vi "Initialise Teapot.vi"(8 "error in (no error)":errorcluster, 11 "Resource Directory":path) -> (0 "error out":errorcluster, 3 "Teapot":T1 {"Triangles"."Vertex 3"."UV"."v" min=0 max=1 step=0.1; "Triangles"."Vertex 3"."UV"."u" min=0 max=1 step=0.1; "Triangles"."Vertex 2"."UV"."v" min=0 max=1 step=0.1; "Triangles"."Vertex 2"."UV"."u" min=0 max=1 step=0.1; "Triangles"."Vertex 1"."UV"."v" min=0 max=1 step=0.1; "Triangles"."Vertex 1"."UV"."u" min=0 max=1 step=0.1})   [LabVIEW 2022 SP3, in "Application.lvlib" / "Scene.lvclass"]
uses:
  Scene.lvclass
  Libraries/3D/Object.ctl
  Libraries/3D/Vector 3D.ctl
  Libraries/3D/Transform.ctl
  <userlib>/_OpenG.lib/file/file.llb/Convert File Extension (Path)__ogtk.vi
  Scene.lvclass/Scene.ctl
  Libraries/3D/3D.lvlib
  Libraries/Raster/UV.ctl
  Libraries/Raster/Raster.lvlib
  Libraries/3D/Vertex.ctl
  Libraries/3D/Triangle.ctl
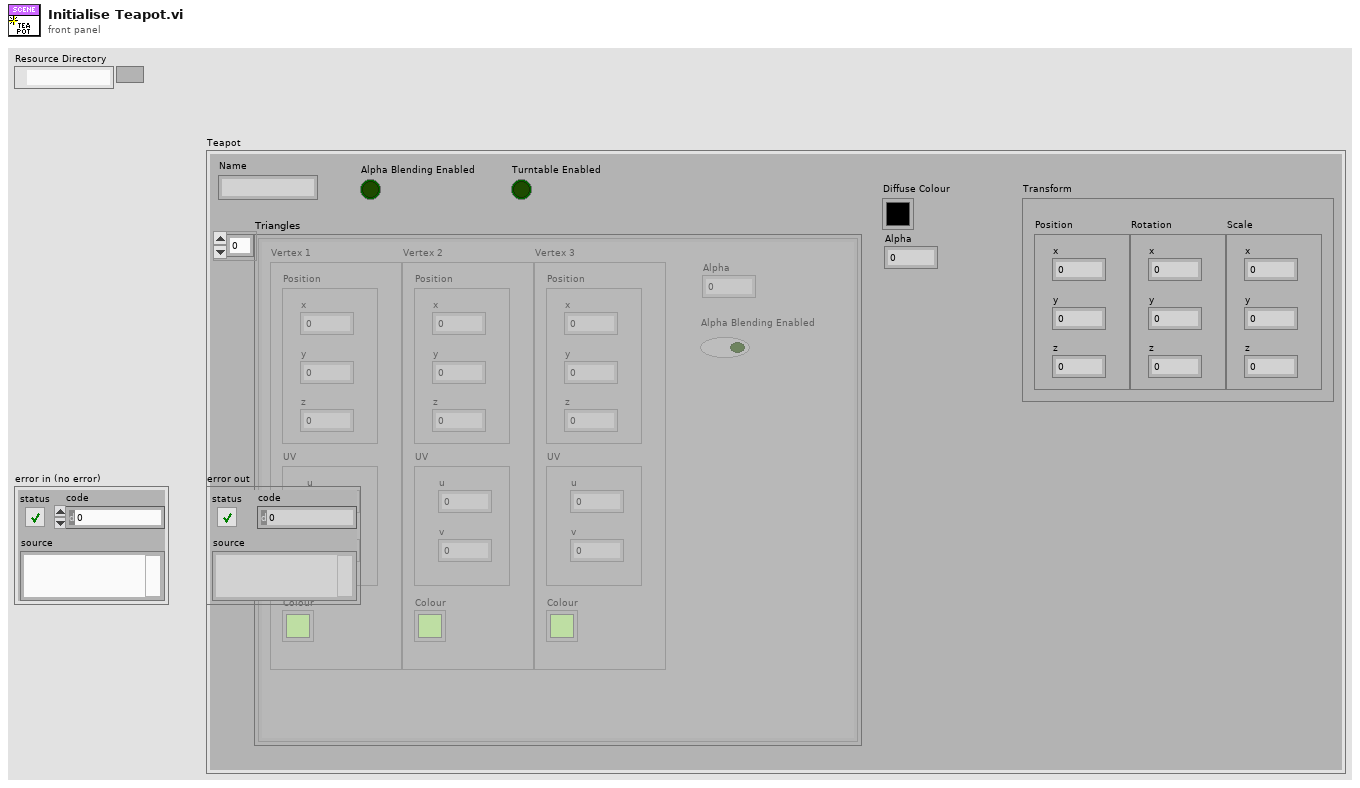
[diagram p1: front panel]
types:
  T1 = typedef "3D.lvlib/Object.ctl" = cluster{"Triangles":T2[], "Diffuse Colour":u32, "Transform":T6, "Name":string, "Alpha Blending Enabled":bool, "Alpha":dbl, "Turntable Enabled":bool}
  T2 = typedef "3D.lvlib/Triangle.ctl" = cluster{"Vertex 1":T3, "Vertex 2":T3, "Vertex 3":T3, "Alpha":dbl, "Alpha Blending Enabled":bool}
  T3 = typedef "3D.lvlib/Vertex.ctl" = cluster{"Position":T4, "UV":T5, "Colour":u32}
  T4 = typedef "3D.lvlib/Vector 3D.ctl" = cluster{"x":sgl, "y":sgl, "z":sgl}
  T5 = typedef "Raster.lvlib/UV.ctl" = cluster{"u":sgl, "v":sgl}
  T6 = typedef "3D.lvlib/Transform.ctl" = cluster{"Position":T4, "Rotation":T4, "Scale":T4}
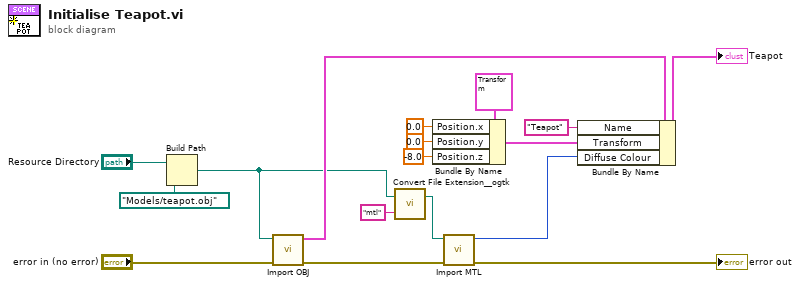
[diagram p0: block diagram]
diagram:
  n1 = Build Path(base path="Resource Directory", name or relative path=path "Models/teapot.obj") -> (appended path=w3:path)
  n2 = call "Import OBJ.vi"("error in (no error)"="error in (no error)", "Object"=w3) -> ("error out"=w2:errorcluster, "Object"=w5:T1)  [unwired: 8 in]
  n3 = call-poly <userlib>:"Convert File Extension__ogtk.vi"("new ending (none)"="mtl", "file name"=w3) -> ("new filename"=w8:path)  [unwired: 1 out]
  n4 = Bundle By Name(cluster=T6 {"Position"={"x"=2.0, "y"=1.0, "z"=-5.0}, "Rotation"={"x"=0.0, "y"=0.0, "z"=0.0}, "Scale"={"x"=0.0, "y"=0.0, "z"=0.0}} ("Transform"), "Position.x"=sgl 0.0, "Position.y"=sgl 0.0, "Position.z"=sgl -8.0) -> (w11:T6)
  n5 = call "Import MTL.vi"("error in (no error)"=w2, "Material"=w8) -> ("error out"=→"error out":errorcluster, "Diffuse Colour"=w6:u32)  [unwired: 8 in]
  n6 = Bundle By Name(cluster=w5, "Name"="Teapot", "Transform"=w11, "Diffuse Colour"=w6) -> (→"Teapot":T1)
